vi "Read GroupName.vi"(8 "error in":errorcluster, 11 "group in":refnum<class "_Group.lvclass">) -> (0 "error out":errorcluster, 2 "groupName":string, 3 "group out":refnum<class "_Group.lvclass">)   [LabVIEW 2013, in "_Group.lvclass"]
uses:
  _Group.lvclass
  _Group.lvclass/_Group.ctl
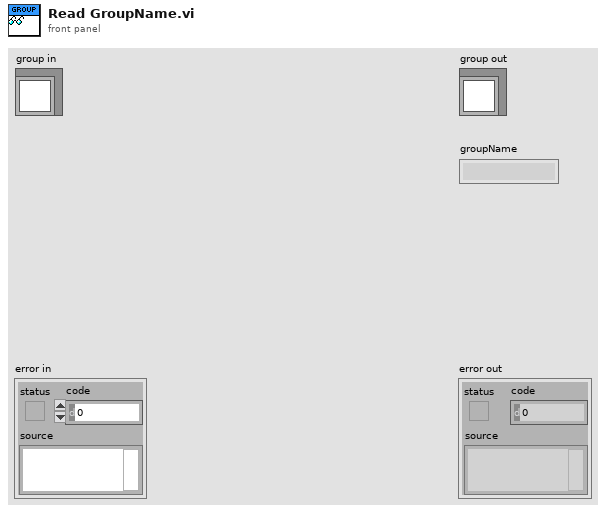
[diagram p1: front panel]
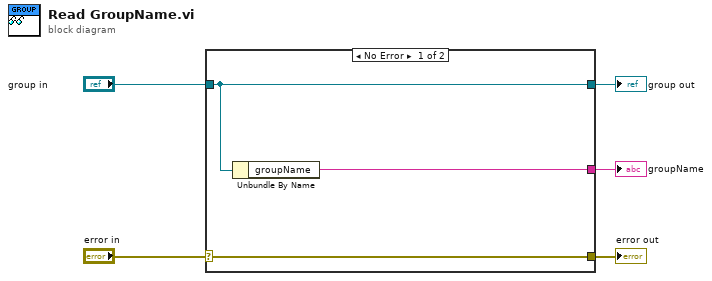
[diagram p0: block diagram]
diagram:
  n1 = case shown="No Error" "error in" {
    selector: "error in" -> [w8 w9]
    tunnel: [w8 w9] -> w4
    tunnel: [w7 w10] -> w2
    tunnel: "group in" -> [w7 w10]
    tunnel: [w6 _] -> w1
    frame No Error {
      n2 = Unbundle By Name(w7) -> ("groupName"=w6:string)
    }
    frame Error {
    }
  }
  "error out" <- w4
  "group out" <- w2
  "groupName" <- w1
